vi "Add Binding.vi"(8 "error in (no error)":errorcluster, 9 "Sink":refnum<class "Binding.lvclass">, 10 "Source":refnum<class "Binding.lvclass">, 11 "MultiBinding in (New)":refnum<class "MultiBinding.lvclass">) -> (0 "error out":errorcluster, 3 "MultiBinding out":refnum<class "MultiBinding.lvclass">)   [LabVIEW 2020, in "PropertyBinder.lvlib" / "MultiBinding.lvclass"]
uses:
  MultiBinding.lvclass
  Binding/Binding.lvclass
  MultiBinding.lvclass/MultiBinding.ctl
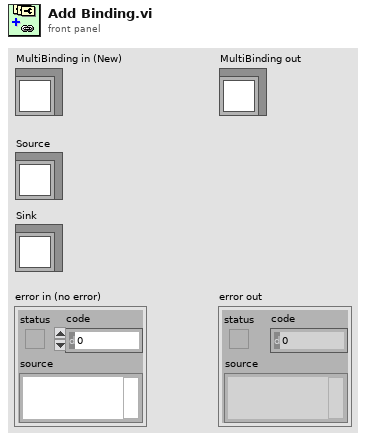
[diagram p1: front panel]
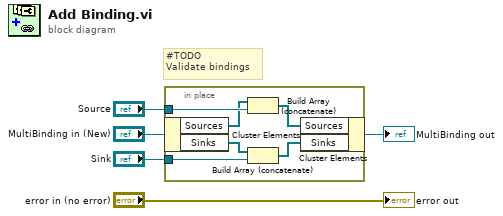
[diagram p0: block diagram]
diagram:
  # "#TODO\nValidate bindings"
  n1 = in-place {
    in-place-border: "Sink" -> [w7]
    in-place-border: "Source" -> [w11]
    n2 = in-place-cluster #1("MultiBinding in (New)") -> ("Sources"=w10:refnum<class "Binding.lvclass">[], "Sinks"=w8:refnum<class "Binding.lvclass">[])
    n3 = Build Array (concatenate)(w10, w11) -> (w9:refnum<class "Binding.lvclass">[])
    n4 = Build Array (concatenate)(w8, w7) -> (w6:refnum<class "Binding.lvclass">[])
    n5 = in-place-cluster #1("Sources"=w9, "Sinks"=w6) -> (→"MultiBinding out":refnum<class "MultiBinding.lvclass">)
  }
  "error out" <- "error in (no error)"
